vi "broadcastHPFreezeSensorValues.vi"(8 "error in (no error)":errorcluster, 9 "Subnet":u8, 10 "ModbusBuffer in":refnum<class "ModbusBuffer.lvclass">, 11 "ILCCommunications in":refnum<class "ILCCommunications.lvclass">) -> (0 "error out":errorcluster, 2 "ModbusBuffer out":refnum<class "ModbusBuffer.lvclass">, 3 "ILCCommunications out":refnum<class "ILCCommunications.lvclass">)   [LabVIEW 2016, in "ILCCommunications.lvclass"]
uses:
  ILCCommunications.lvclass
  Common_RT_Modbus/ModbusBuffer/ModbusBuffer.lvclass
  ILCCommunications.lvclass/ILCCommunications.ctl
  Common_RT_HPILC/HPILC/HPILC.lvclass/HPILC.ctl
  Common_RT_Modbus/ModbusBuffer/ModbusBuffer.lvclass/ModbusBuffer.ctl
  Common_RT_Modbus/ModbusBuffer/writeHeader.vi
  Common_RT_Modbus/ModbusBuffer/writeU8.vi
  Common_RT_Modbus/ModbusBuffer/writeCRC.vi
  Common_RT_Modbus/ModbusBuffer/writeDelay.vi
  Common_RT_Modbus/ModbusBuffer/writeEndOfFrame.vi
  Common_RT_Modbus/ModbusBuffer/writeByteInstruction.vi
  Common_RT_Modbus/ModbusBuffer/calculateCRC.vi
  Common_RT_HPILC/HPILC/HPILC.lvclass
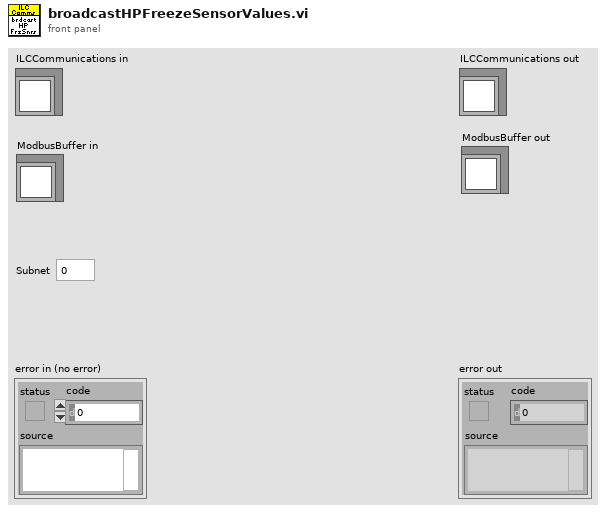
[diagram p1: front panel]
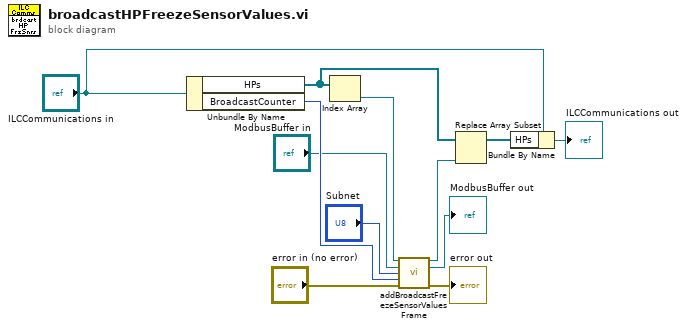
[diagram p0: block diagram]
diagram:
  n1 = Unbundle By Name("ILCCommunications in") -> ("HPs"=w8:refnum<class "HPILC.lvclass">[], "BroadcastCounter"=w12:u8)
  n2 = Index Array(array=w8) -> (element=w11:refnum<class "HPILC.lvclass">)  [unwired: 1 in]
  n3 = call "addBroadcastFreezeSensorValuesFrame.vi"("HPILC in"=w11, "ModbusBuffer in"="ModbusBuffer in", "Subnet"="Subnet", "BroadcastCounter"=w12, "error in (no error)"="error in (no error)") -> ("HPILC out"=w7:refnum<class "HPILC.lvclass">, "ModbusBuffer out"=→"ModbusBuffer out":refnum<class "ModbusBuffer.lvclass">, "error out"=→"error out":errorcluster)  [unwired: 8 in]
  n4 = Replace Array Subset(array=w8, new element=w7) -> (w4:refnum<class "HPILC.lvclass">[])  [unwired: 1 in]
  n5 = Bundle By Name(cluster="ILCCommunications in", "HPs"=w4) -> (→"ILCCommunications out":refnum<class "ILCCommunications.lvclass">)
